vi "Finish.vi"   [LabVIEW 2012]
doc: "This VI is called just before exiting. It is expected to close I/O refnum, save collected data, etc."
uses:
  <vilib>/Rock Robotics/WPI/Compressor/WPI_CompressorGetSetRefNum.vi
  <vilib>/Rock Robotics/WPI/Joystick/WPI_JoystickGetSetRefNum.vi
  <vilib>/Rock Robotics/WPI/RobotDrive/WPI_RobotDriveGetSetRefNum.vi
types:
  T1 = typedef "WPI_MotorControlDeviceRef.ctl" = cluster{"DeviceStatus":errorcluster, "Type":enum16{"PWM", "CAN"}, "PWM":cluster{"Digital Module":T2, "PWM Channel":T3, "DeadBand":T4}, "CAN":cluster{"Device Number":u8, "Control Mode":T5, "Semaphore":T6, "Max Vout":dbl}, "Invert":bool, "TransformRef":T7, "InvTransformRef":T7}
  T2 = typedef "FPGA_TypedefDigitalModule.ctl" = enum16{"Digital Module 1", "Digital Module 2"}
  T3 = typedef "FPGA_DIOPWMChannel.ctl" = enum8{"PWM 1", "PWM 2", "PWM 3", "PWM 4", "PWM 5", "PWM 6", "PWM 7", "PWM 8", "PWM 9", "PWM 10", "Invalid"}
  T4 = typedef "WPI_PWMDeadband.ctl" = cluster{"Name":string, "maxPositivePwm":i32, "minPositivePwm":i32, "centerPwm":i32, "maxNegativePwm":i32, "minNegativePwm":i32, "angularRange":u16}
  T5 = typedef "WPI_CANJaguar_ControlMode.ctl" = enum8{"Percent VBus", "Current", "Speed", "Position", "Voltage"}
  T6 = typedef "Semaphore RefNum" = refnum<k1>
  T7 = typedef "WPI_PWMTransform_ConPane.ctl" = refnum<vi>
  T8 = typedef "WPI_DigitalInputDevRef.ctl" = cluster{"DevStatus":errorcluster, "DIO Channel":T9, "Digital Module":T2}
  T9 = typedef "FPGA_DIOChannel.ctl" = enum8{"DIO 1", "DIO 2", "DIO 3", "DIO 4", "DIO 5", "DIO 6", "DIO 7", "DIO 8", "DIO 9", "DIO 10", "DIO 11", "DIO 12", "DIO 13", "DIO 14", "Invalid"}
  T10 = typedef "WPI_JoystickDevRef.ctl" = cluster{"Device":T11}
  T11 = typedef "WPI_JoystickDeviceEnum.ctl" = enum16{"USB 1", "USB 2", "USB 3", "USB 4", "Kinect 1", "Kinect 2"}
  T12 = typedef "WPI_RobotDriveDevRef.ctl" = cluster{"DevStatus":errorcluster, "Motors[]":T1[], "Square Inputs":bool, "Max Output":dbl, "Isochronous":bool}
  T13 = typedef "WPI_SolenoidDevRef.ctl" = cluster{"DevStatus":errorcluster, "Solenoid Module":T14, "Forward Solenoid Channel":T15, "Reverse Solenoid Channel":T15}
  T14 = typedef "FPGA_TypedefSolenoidModule.ctl" = enum16{"Solenoid Module 1", "Solenoid Module 2"}
  T15 = typedef "WPI_SolenoidChannel.ctl" = enum8{"Solenoid 1", "Solenoid 2", "Solenoid 3", "Solenoid 4", "Solenoid 5", "Solenoid 6", "Solenoid 7", "Solenoid 8", "Invalid"}
  T16 = typedef "WPI_EncoderDevRef.ctl" = cluster{"DevStatus":errorcluster, "EncoderIndex":T17, "CounterIndex":T18, "DistancePerCount":dbl, "Decoding Type":T19}
  T17 = typedef "FPGA_EncoderIdx.ctl" = enum8{"Enc 0", "Enc 1", "Enc 2", "Enc 3", "Invalid"}
  T18 = typedef "FPGA_CounterCtrSystemIndex.ctl" = enum8{"Ctr 0", "Ctr 1", "Ctr 2", "Ctr 3", "Ctr 4", "Ctr 5", "Ctr 6", "Ctr 7", "Invalid"}
  T19 = typedef "WPI_EncoderType.ctl" = enum16{"1x", "2x", "4x"}
  T20 = typedef "WPI_GyroDevRef.ctl" = cluster{"DevStatus":errorcluster, "Analog Module":T21, "Analog Channel":T22, "Offset":dbl, "Gain (VoltsPerDegree/Second)":dbl}
  T21 = typedef "FPGA_TypedefAnalogModule.ctl" = enum16{"Analog Module 1", "Analog Module 2"}
  T22 = typedef "FPGA_AIChannel.ctl" = enum8{"AI 1", "AI 2", "AI 3", "AI 4", "AI 5", "AI 6", "AI 7", "AI 8", "Invalid"}
  T23 = typedef "WPI_CompressorDevRef.ctl" = cluster{"DevStatus":errorcluster, "DigitalInputDevRef":T8, "RelayDevRef":T24}
  T24 = typedef "WPI_RelayDevRef.ctl" = cluster{"DevStatus":errorcluster, "Relay Channel":T25, "Digital Module":T2, "Relay Direction":T26}
  T25 = typedef "FPGA_DIORelayChannel.ctl" = enum8{"Relay 1", "Relay 2", "Relay 3", "Relay 4", "Relay 5", "Relay 6", "Relay 7", "Relay 8", "Invalid"}
  T26 = typedef "WPI_RelayDirection.ctl" = enum16{"Both directions", "Forward only", "Reverse only"}
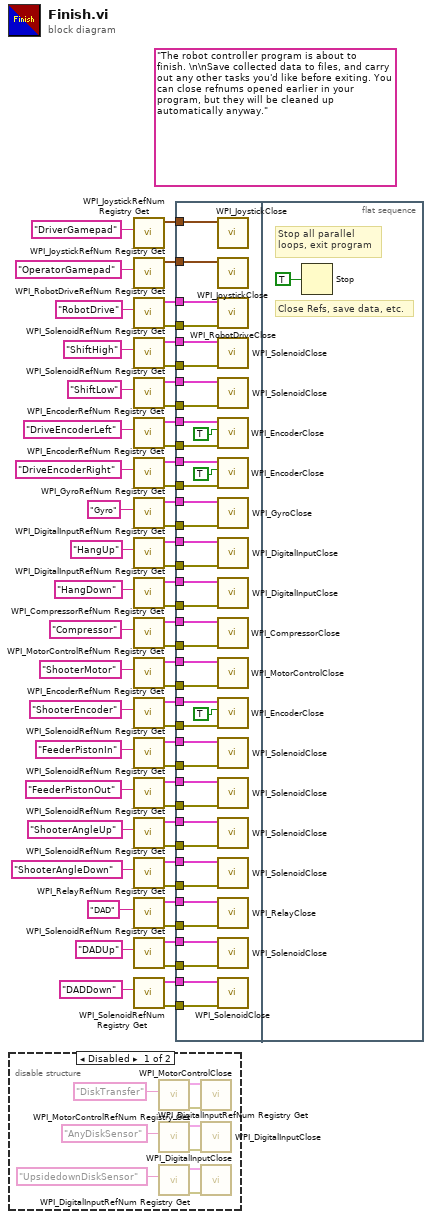
[diagram p0: block diagram]
diagram:
  (unwired) "The robot controller program is about to finish. \n\nSave collected data to files, and carry out any other tasks you'd like before exiting. You can close refnums opened earlier in your program, but they will be cleaned up automatically anyway."
  n1 = disable-structure shown="Disabled" {
    frame Disabled {
      n2 = call <vilib>:"WPI_MotorControlRefNum Registry Get.vi"("refnum name"="DiskTransfer") -> ("error out"=w63:errorcluster, "MotorControlDevRef"=w64:T1)  [unwired: 9 in]
      n3 = call <vilib>:"WPI_DigitalInputRefNum Registry Get.vi"("refnum name"="AnyDiskSensor") -> ("error out"=w61:errorcluster, "DigitalInputDevRef"=w62:T8)  [unwired: 9 in]
      n4 = call <vilib>:"WPI_DigitalInputRefNum Registry Get.vi"("refnum name"="UpsidedownDiskSensor") -> ("error out"=w59:errorcluster, "DigitalInputDevRef"=w60:T8)  [unwired: 9 in]
      n5 = call <vilib>:"WPI_MotorControlClose.vi"("error in (no error)"=w63, "MotorControlDevRef"=w64) -> ()  [unwired: 9 in, 1 out]
      n6 = call <vilib>:"WPI_DigitalInputClose.vi"("error in (no error)"=w61, "DigitalInputDevRef"=w62) -> ()  [unwired: 9 in, 1 out]
      n7 = call <vilib>:"WPI_DigitalInputClose.vi"("error in (no error)"=w59, "DigitalInputDevRef"=w60) -> ()  [unwired: 9 in, 1 out]
    }
    frame Enabled {
    }
  }
  n8 = call <vilib>:"WPI_JoystickRefNum Registry Get.vi"("refnum name"="DriverGamepad") -> ("JoystickDevRef"=w38:T10)  [unwired: 1 in, 9 out]
  n9 = call <vilib>:"WPI_JoystickRefNum Registry Get.vi"("refnum name"="OperatorGamepad") -> ("JoystickDevRef"=w37:T10)  [unwired: 1 in, 9 out]
  n10 = call <vilib>:"WPI_RobotDriveRefNum Registry Get.vi"("refnum name"="RobotDrive") -> ("error out"=w34:errorcluster, "RobotDriveDevRef"=w36:T12)  [unwired: 1 in, 8 out]
  n11 = call <vilib>:"WPI_SolenoidRefNum Registry Get.vi"("refnum name"="ShiftHigh") -> ("error out"=w33:errorcluster, "SolenoidDevRef"=w35:T13)  [unwired: 9 in]
  n12 = call <vilib>:"WPI_SolenoidRefNum Registry Get.vi"("refnum name"="ShiftLow") -> ("error out"=w31:errorcluster, "SolenoidDevRef"=w32:T13)  [unwired: 9 in]
  n13 = call <vilib>:"WPI_EncoderRefNum Registry Get.vi"("refnum name"="DriveEncoderLeft") -> ("error out"=w29:errorcluster, "EncoderDevRef"=w30:T16)  [unwired: 9 in]
  n14 = call <vilib>:"WPI_EncoderRefNum Registry Get.vi"("refnum name"="DriveEncoderRight") -> ("error out"=w25:errorcluster, "EncoderDevRef"=w26:T16)  [unwired: 9 in]
  n15 = call <vilib>:"WPI_GyroRefNum Registry Get.vi"("refnum name"="Gyro") -> ("error out"=w27:errorcluster, "GyroDevRef"=w28:T20)  [unwired: 9 in]
  n16 = call <vilib>:"WPI_DigitalInputRefNum Registry Get.vi"("refnum name"="HangUp") -> ("error out"=w23:errorcluster, "DigitalInputDevRef"=w24:T8)  [unwired: 9 in]
  n17 = call <vilib>:"WPI_DigitalInputRefNum Registry Get.vi"("refnum name"="HangDown") -> ("error out"=w21:errorcluster, "DigitalInputDevRef"=w22:T8)  [unwired: 9 in]
  n18 = call <vilib>:"WPI_CompressorRefNum Registry Get.vi"("refnum name"="Compressor") -> ("error out"=w19:errorcluster, "CompressorDevRef"=w20:T23)  [unwired: 9 in]
  n19 = call <vilib>:"WPI_MotorControlRefNum Registry Get.vi"("refnum name"="ShooterMotor") -> ("error out"=w17:errorcluster, "MotorControlDevRef"=w18:T1)  [unwired: 9 in]
  n20 = call <vilib>:"WPI_EncoderRefNum Registry Get.vi"("refnum name"="ShooterEncoder") -> ("error out"=w15:errorcluster, "EncoderDevRef"=w16:T16)  [unwired: 9 in]
  n21 = call <vilib>:"WPI_SolenoidRefNum Registry Get.vi"("refnum name"="FeederPistonIn") -> ("error out"=w13:errorcluster, "SolenoidDevRef"=w14:T13)  [unwired: 9 in]
  n22 = call <vilib>:"WPI_SolenoidRefNum Registry Get.vi"("refnum name"="FeederPistonOut") -> ("error out"=w11:errorcluster, "SolenoidDevRef"=w12:T13)  [unwired: 9 in]
  n23 = call <vilib>:"WPI_SolenoidRefNum Registry Get.vi"("refnum name"="ShooterAngleUp") -> ("error out"=w9:errorcluster, "SolenoidDevRef"=w10:T13)  [unwired: 9 in]
  n24 = call <vilib>:"WPI_SolenoidRefNum Registry Get.vi"("refnum name"="ShooterAngleDown") -> ("error out"=w7:errorcluster, "SolenoidDevRef"=w8:T13)  [unwired: 9 in]
  n25 = call <vilib>:"WPI_RelayRefNum Registry Get.vi"("refnum name"="DAD") -> ("error out"=w5:errorcluster, "RelayDevRef"=w6:T24)  [unwired: 9 in]
  n26 = call <vilib>:"WPI_SolenoidRefNum Registry Get.vi"("refnum name"="DADUp") -> ("error out"=w3:errorcluster, "SolenoidDevRef"=w4:T13)  [unwired: 9 in]
  n27 = call <vilib>:"WPI_SolenoidRefNum Registry Get.vi"("refnum name"="DADDown") -> ("error out"=w1:errorcluster, "SolenoidDevRef"=w2:T13)  [unwired: 9 in]
  n28 = flat-sequence {
    tunnel: w38 -> [w108]
    tunnel: w37 -> [w107]
    tunnel: w36 -> [w106]
    tunnel: w35 -> [w105]
    tunnel: w34 -> [w104]
    tunnel: w33 -> [w103]
    tunnel: w32 -> [w102]
    tunnel: w31 -> [w101]
    tunnel: w30 -> [w100]
    tunnel: w29 -> [w99]
    tunnel: w28 -> [w95]
    tunnel: w27 -> [w94]
    tunnel: w26 -> [w93]
    tunnel: w25 -> [w92]
    tunnel: w24 -> [w91]
    tunnel: w23 -> [w90]
    tunnel: w22 -> [w89]
    tunnel: w21 -> [w88]
    tunnel: w20 -> [w87]
    tunnel: w19 -> [w86]
    tunnel: w18 -> [w85]
    tunnel: w17 -> [w84]
    tunnel: w16 -> [w83]
    tunnel: w15 -> [w82]
    tunnel: w14 -> [w81]
    tunnel: w13 -> [w80]
    tunnel: w12 -> [w79]
    tunnel: w11 -> [w78]
    tunnel: w10 -> [w77]
    tunnel: w9 -> [w76]
    tunnel: w8 -> [w75]
    tunnel: w7 -> [w74]
    tunnel: w6 -> [w73]
    tunnel: w5 -> [w72]
    tunnel: w4 -> [w71]
    tunnel: w3 -> [w70]
    tunnel: w2 -> [w69]
    tunnel: w1 -> [w68]
    frame #0 {
      n29 = call <vilib>:"WPI_JoystickClose.vi"("JoystickDevRef"=w108) -> ()  [unwired: 11 out]
      n30 = call <vilib>:"WPI_JoystickClose.vi"("JoystickDevRef"=w107) -> ()  [unwired: 11 out]
      n31 = call <vilib>:"WPI_RobotDriveClose.vi"("error in (no error)"=w104, "RobotDriveDevRef"=w106) -> ()  [unwired: 10 out]
      n32 = call <vilib>:"WPI_SolenoidClose.vi"("error in (no error)"=w103, "SolenoidDevRef"=w105) -> ()  [unwired: 9 in, 1 out]
      n33 = call <vilib>:"WPI_SolenoidClose.vi"("error in (no error)"=w101, "SolenoidDevRef"=w102) -> ()  [unwired: 9 in, 1 out]
      n34 = call <vilib>:"WPI_EncoderClose.vi"("error in (no error)"=w99, "Close Dependencies"=TRUE, "EncoderDevRef"=w100) -> ()  [unwired: 8 in, 1 out]
      n35 = call <vilib>:"WPI_EncoderClose.vi"("error in (no error)"=w92, "Close Dependencies"=TRUE, "EncoderDevRef"=w93) -> ()  [unwired: 8 in, 1 out]
      n36 = call <vilib>:"WPI_GyroClose.vi"("error in (no error)"=w94, "GyroDevRef"=w95) -> ()  [unwired: 9 in, 1 out]
      n37 = call <vilib>:"WPI_DigitalInputClose.vi"("error in (no error)"=w90, "DigitalInputDevRef"=w91) -> ()  [unwired: 9 in, 1 out]
      n38 = call <vilib>:"WPI_DigitalInputClose.vi"("error in (no error)"=w88, "DigitalInputDevRef"=w89) -> ()  [unwired: 9 in, 1 out]
      n39 = call <vilib>:"WPI_CompressorClose.vi"("error in (no error)"=w86, "CompressorDevRef"=w87) -> ()  [unwired: 9 in, 1 out]
      n40 = call <vilib>:"WPI_MotorControlClose.vi"("error in (no error)"=w84, "MotorControlDevRef"=w85) -> ()  [unwired: 9 in, 1 out]
      n41 = call <vilib>:"WPI_EncoderClose.vi"("error in (no error)"=w82, "Close Dependencies"=TRUE, "EncoderDevRef"=w83) -> ()  [unwired: 8 in, 1 out]
      n42 = call <vilib>:"WPI_SolenoidClose.vi"("error in (no error)"=w80, "SolenoidDevRef"=w81) -> ()  [unwired: 9 in, 1 out]
      n43 = call <vilib>:"WPI_SolenoidClose.vi"("error in (no error)"=w78, "SolenoidDevRef"=w79) -> ()  [unwired: 9 in, 1 out]
      n44 = call <vilib>:"WPI_SolenoidClose.vi"("error in (no error)"=w76, "SolenoidDevRef"=w77) -> ()  [unwired: 9 in, 1 out]
      n45 = call <vilib>:"WPI_SolenoidClose.vi"("error in (no error)"=w74, "SolenoidDevRef"=w75) -> ()  [unwired: 9 in, 1 out]
      n46 = call <vilib>:"WPI_RelayClose.vi"("error in (no error)"=w72, "RelayDevRef"=w73) -> ()  [unwired: 9 in, 1 out]
      n47 = call <vilib>:"WPI_SolenoidClose.vi"("error in (no error)"=w70, "SolenoidDevRef"=w71) -> ()  [unwired: 9 in, 1 out]
      n48 = call <vilib>:"WPI_SolenoidClose.vi"("error in (no error)"=w68, "SolenoidDevRef"=w69) -> ()  [unwired: 9 in, 1 out]
    }
    frame #1 {
      # "Close Refs, save data, etc."
      # "Stop all parallel\nloops, exit program"
      n49 = Stop(stop? (T)=TRUE ("Quit")) -> ()
    }
  }
